vi "Left.vi"(1 "背景":dbl[][](array[numeric]), 2 "方块":dbl[][](array[numeric]), 3 "point":cluster{"x":i16, "y":i16} caption="位置") -> (0 "point 2":cluster{"x":i16, "y":i16} caption="新位置")   [LabVIEW 2016]
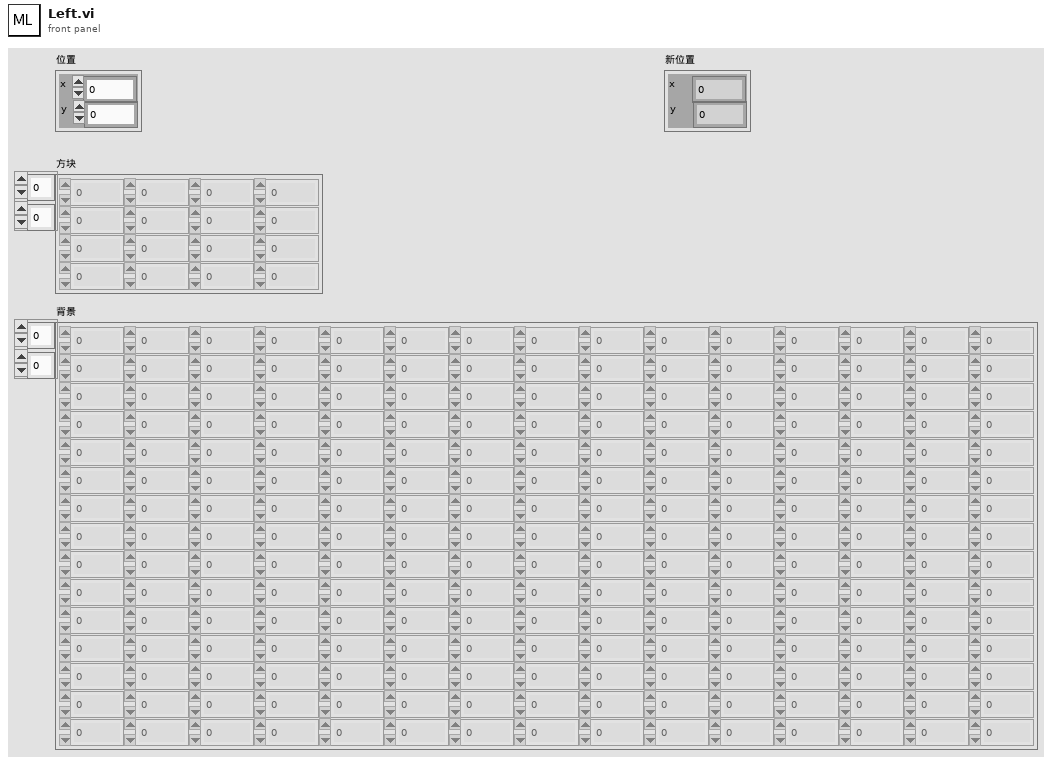
[diagram p1: front panel]
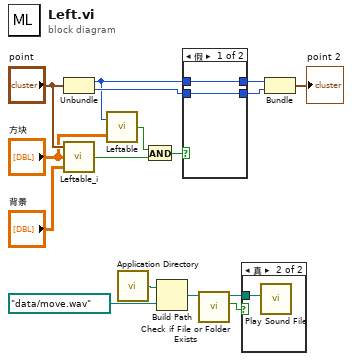
[diagram p0: block diagram]
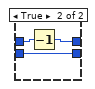
[diagram p3: hidden frame]
diagram:
  n1 = Unbundle("point") -> ("x"=w11:i16, "y"=w15:i16)
  n2 = call "Leftable_i.vi"("背景"="背景", "方块"="方块", "point"="point") -> ("输出"=w7:bool)
  n3 = call "Leftable.vi"("方块"="方块", "x"=w11) -> ("输出"=w6:bool)
  n4 = call <vilib>:"Application Directory.vi"() -> ("Application Directory"=w4:path)
  n5 = And(x=w6, y=w7) -> (x .and. y?=w16:bool)
  n6 = Build Path(base path=w4, name or relative path=path "data/move.wav") -> (appended path=w3:path)
  n7 = case shown="假" w16 {
    tunnel: w15 -> [w17 w21]
    tunnel: w11 -> [w18 w19]
    tunnel: [w18 w20] -> w14
    tunnel: [w17 w21] -> w13
    frame False {
    }
    frame True {
      n8 = Decrement(x=w19) -> (x-1=w20:i16)
    }
  }
  n9 = call <vilib>:"Check if File or Folder Exists.vi"("path"=w3) -> ("file or folder exists?"=w2:bool, "dup path"=w1:path)  [unwired: 8 in, 1 out]
  n10 = case shown="真" w2 {
    tunnel: w1 -> [_ w22]
    frame False {
    }
    frame True {
      n11 = call <vilib>:"Play Sound File.vi"("path"=w22) -> ()  [unwired: 9 in, 2 out]
    }
  }
  n12 = Bundle("x"=w14, "y"=w13) -> (→"point 2":cluster{"x":i16, "y":i16})  [unwired: 1 in]
